vi "myRIO_BRig_RT_arrTrig_init.vi"() -> (3 "output_arrTrig":bool[](array[boolean]))   [LabVIEW 2014]
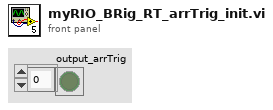
[diagram p1: front panel]
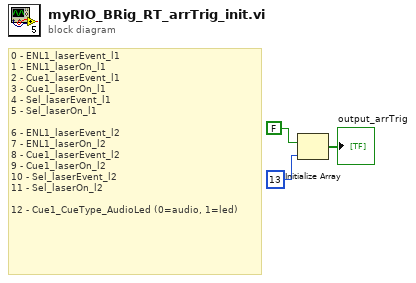
[diagram p0: block diagram]
diagram:
  # "0 - ENL1_laserEvent_l1\n1 - ENL1_laserOn_l1\n2 - Cue1_laserEvent_l1\n3 - Cue1_laserOn_l1\n4 - Sel_laserEvent_l1\n5 - Sel_laserOn_l1\n\n6 - ENL1_laserEvent_l2\n7 - ENL1_laserOn_l2\n8 - Cue1_laserEvent_l2\n9 - Cue1_laserOn_l2\n10 - Sel_laserEvent_l2\n11 - Sel_laserOn_l2\n\n12 - Cue1_CueType_AudioLed (0=audio, 1=led)"
  n1 = Initialize Array(FALSE, 13 ("dimension size")) -> (→"output_arrTrig":bool[])
